vi "Load-CryptoNight-Step3.vi"(8 "error in":errorcluster, 11 "FileName":string="log_file.8.bin") -> (0 "error out":errorcluster, 3 "output cluster":T1)   [LabVIEW 2017]
panel:
  out "b":u64[](array[numeric]) format="%.0x"
  out "hp_state_out":u8[](array[numeric]) format="%.0x"
  out "a":u64[](array[numeric]) format="%.0x"
  out "hp_state_in":u8[](array[numeric]) format="%.0x"
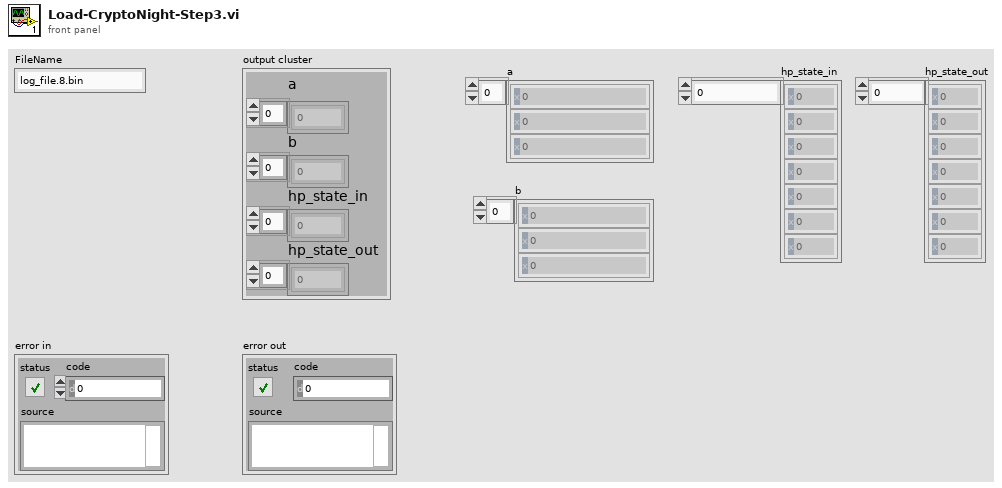
[diagram p1: front panel]
types:
  T1 = cluster{"a":u64[], "b":u64[], "hp_state_in":u8[], "hp_state_out":u8[]}
  T2 = enum16{"big-endian, network order", "native, host order", "little-endian"}
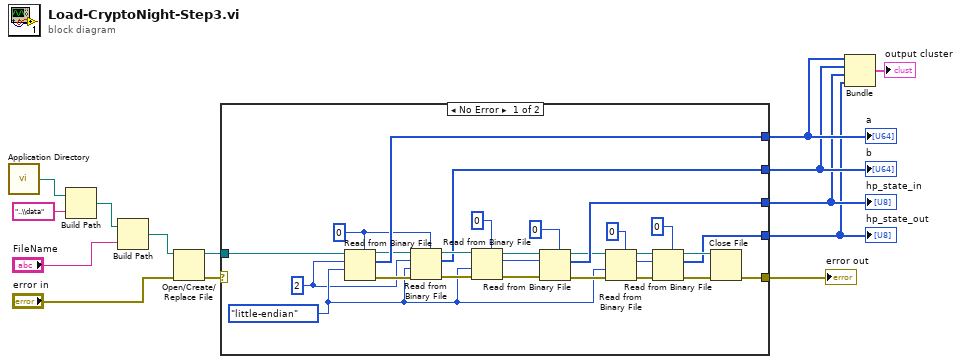
[diagram p0: block diagram]
diagram:
  n1 = call <vilib>:"Application Directory.vi"() -> ("Application Directory"=w6:path)
  n2 = Build Path(base path=w6, name or relative path="..\\data") -> (appended path=w14:path)
  n3 = Build Path(base path=w14, name or relative path="FileName") -> (appended path=w7:path)
  n4 = Open/Create/Replace File(file path (use dialog)=w7, error in="error in") -> (refnum out=w8:refnum<file>, error out=w9:errorcluster)  [unwired: 4 in, 1 out]
  n5 = case shown="No Error" w9 {
    selector: w9 -> [_ w42]
    tunnel: [w38 _] -> w3
    tunnel: [w41 w42] -> w11
    tunnel: [w35 _] -> w5
    tunnel: [w29 _] -> w2
    tunnel: w8 -> [w26 _]
    tunnel: [w15 _] -> w4
    frame No Error {
      w16 = 2 ("count (1)")
      w17 = T2."little-endian" ("byte order (0:big-endian, network order)")
      w20 = u64 0
      n6 = Read from Binary File(5:w20, 9:w17, 10:w16, 11:w26) -> (0:w22:errorcluster, 2:w35:u64[], 3:w19:refnum<file>)  [unwired: 2 in, 1 out]
      n7 = Read from Binary File(5:w20, 8:w22, 9:w17, 10:w16, 11:w19) -> (0:w21:errorcluster, 2:w15:u64[], 3:w18:refnum<file>)  [unwired: 1 in, 1 out]
      n8 = Read from Binary File(5:u32 0, 8:w21, 9:w17, 11:w18) -> (0:w39:errorcluster, 2:w23:u32, 3:w36:refnum<file>)  [unwired: 2 in, 1 out]
      n9 = Read from Binary File(5:u8 0, 8:w39, 10:w23, 11:w36) -> (0:w32:errorcluster, 2:w38:u8[], 3:w27:refnum<file>)  [unwired: 2 in, 1 out]
      n10 = Read from Binary File(5:u32 0, 8:w32, 9:w17, 11:w27) -> (0:w33:errorcluster, 2:w25:u32, 3:w24:refnum<file>)  [unwired: 2 in, 1 out]
      n11 = Read from Binary File(5:u8 0, 8:w33, 10:w25, 11:w24) -> (0:w34:errorcluster, 2:w29:u8[], 3:w31:refnum<file>)  [unwired: 2 in, 1 out]
      n12 = Close File(refnum=w31, error in=w34) -> (error out=w41:errorcluster)  [unwired: 1 out]
    }
    frame Error {
    }
  }
  "hp_state_in" <- w3
  "error out" <- w11
  "a" <- w5
  "hp_state_out" <- w2
  "b" <- w4
  n13 = Bundle(w5, w4, w3, w2) -> (→"output cluster":cluster{u64[], u64[], u8[], u8[]})  [unwired: 1 in]
